vi "Save All VI Data.vi"(8 "error in (no error)":errorcluster, 10 "Saved Item Data":refnum<class "Item.lvclass">[](array[class]), 11 "New Item Data":refnum<class "Item.lvclass">[](array[class])) -> (0 "error out":errorcluster, 1 "Items Saved":u32, 2 "Saved Item Data out":refnum<class "Item.lvclass">[](array[class]), 3 "New Item Data out":refnum<class "Item.lvclass">[](array[class]))   [LabVIEW 2020, in "VI Properties Editor.lvlib"]
doc: "Saves all VI data, keeping the new data for any save that did not happen successfully."
uses:
  VI Properties Editor.lvlib
  Classes/Item/Item.lvclass
  <vilib>/LabVIEW Icon API/lv_icon/Classes/Icon/Icon.lvclass
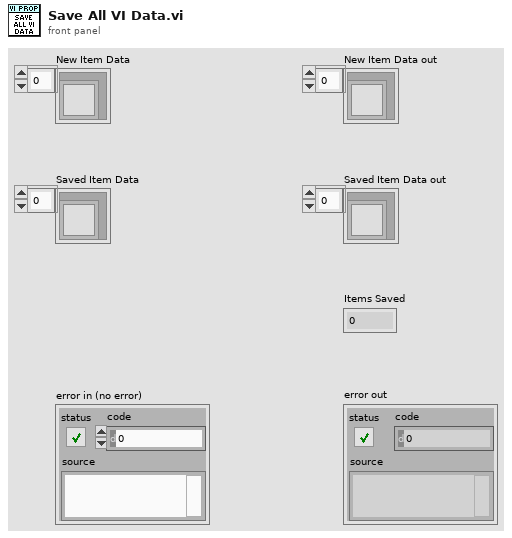
[diagram p1: front panel]
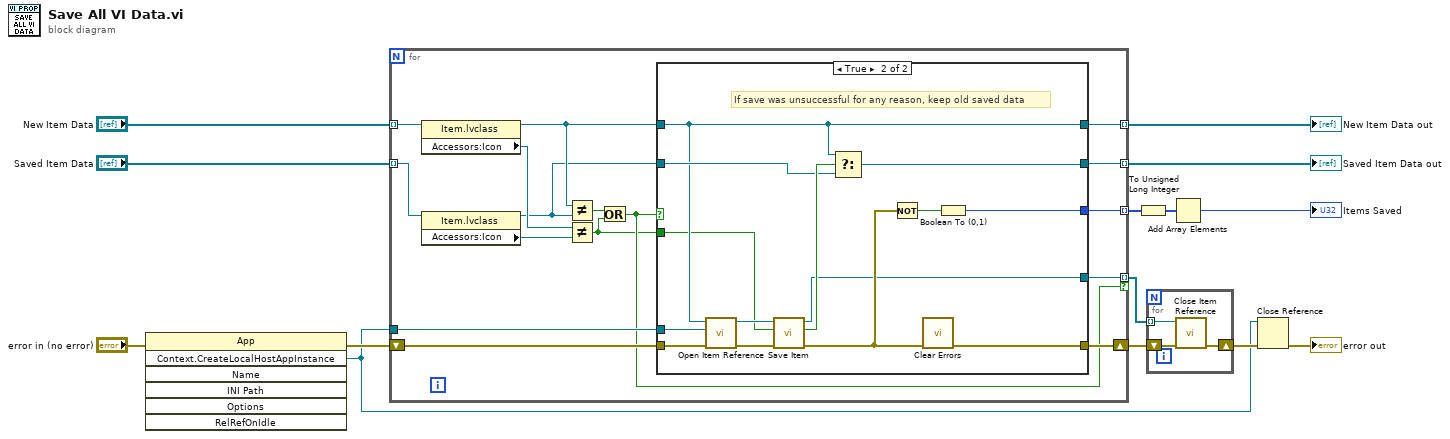
[diagram p0: block diagram]
diagram:
  n1 = invoke class="App" method="Context.CreateLocalHostAppInstance"(error in="error in (no error)") -> (error out=w10:errorcluster, "Create Context"=w9:refnum<vi>)  [unwired: 6 in, 5 out]
  n2 = for {
    shift-right: [w29] -> w14
    shift-left: w10 -> [w30]
    tunnel: "New Item Data" -> [w21] mode=indexing
    tunnel: [w25] -> w4 mode=indexing if=w17
    tunnel: [w27] -> w7 mode=indexing
    tunnel: "Saved Item Data" -> [w20] mode=indexing
    tunnel: [w26] -> w5 mode=indexing
    tunnel: [w16] -> w3 mode=indexing
    tunnel: w9 -> [w28]
    n3 = property class="Item.lvclass"(reference=w21) -> (reference out=w19:refnum<class "Item.lvclass">, "Accessors:Icon"=w22:refnum<class "Icon.lvclass">)  [unwired: 1 in, 1 out]
    n4 = property class="Item.lvclass"(reference=w20) -> (reference out=w18:refnum<class "Item.lvclass">, "Accessors:Icon"=w23:refnum<class "Icon.lvclass">)  [unwired: 1 in, 1 out]
    n5 = Not Equal?(x=w19, y=w18) -> (x != y?=w24:bool)
    n6 = Not Equal?(x=w22, y=w23) -> (x != y?=w15:bool)
    n7 = Or(x=w24, y=w15) -> (x .or. y?=w17:bool)
    n8 = case shown="True" w17 {
      tunnel: w30 -> [w33 w39]
      tunnel: [w33 w47] -> w29
      tunnel: w19 -> [w32 w37]
      tunnel: [w32 w37] -> w27
      tunnel: w18 -> [w31 w44]
      tunnel: [w31 w43] -> w26
      tunnel: [_ w42] -> w25
      tunnel: [_ w40] -> w16
      tunnel: w28 -> [_ w35]
      tunnel: w15 -> [_ w34]
      frame False {
      }
      frame True {
        # "If save was unsuccessful for any reason, keep old saved data"
        n9 = call-dynamic "Open Item Reference.vi"("error in (no error)"=w39, "App Ref (local)"=w35, "Item in"=w37) -> ("error out"=w38:errorcluster, "Item out"=w36:refnum<class "Item.lvclass">)  [unwired: 7 in]
        n10 = call-dynamic "Save Item.vi"("error in (no error)"=w38, "Save Icon?"=w34, "Item in"=w36) -> ("error out"=w46:errorcluster, "Saved?"=w45:bool, "Item out"=w42:refnum<class "Item.lvclass">)  [unwired: 6 in]
        n11 = Select(t=w37, s=w45, f=w44) -> (s? t:f=w43:refnum<class "Item.lvclass">)
        n12 = Not(x=w46) -> (.not. x?=w41:bool)
        n13 = call <vilib>:"Clear Errors.vi"("error in (no error)"=w46) -> ("error out"=w47:errorcluster)  [unwired: 5 in, 1 out]
        n14 = Boolean To (0,1)(Boolean=w41) -> (0, 1=w40:i16)
      }
    }
  }
  "New Item Data out" <- w7
  "Saved Item Data out" <- w5
  n15 = To Unsigned Long Integer(number=w3) -> (unsigned 32bit integer=w1:u32[])
  n16 = for {
    shift-right: [w49] -> w13
    shift-left: w14 -> [w50]
    tunnel: w4 -> [w48] mode=indexing
    n17 = call-dynamic "Close Item Reference.vi"("error in (no error)"=w50, "Item in"=w48) -> ("error out"=w49:errorcluster)  [unwired: 8 in, 1 out]
  }
  n18 = Add Array Elements(numeric array=w1) -> (sum=→"Items Saved":u32)
  n19 = Close Reference(reference=w9, error in (no error)=w13) -> (error out=→"error out":errorcluster)
